vi "Begin.vi"(8 "error in":errorcluster) -> (0 "error out":errorcluster)   [LabVIEW 2015]
doc: "Called before other user functions, this VI is expected to open initial I/O refnums, load in file data, and do all program initialization. Notice that the <B>error out</B> terminal is simply used for data flow. Wiring it to other structures or subVIs ensures that this VI runs first."
uses:
  <vilib>/Rock Robotics/WPI/DriverStation/WPI_DriverStationRobotMode2.ctl
  <vilib>/Rock Robotics/WPI/Joystick/WPI_JoystickDeviceEnum.ctl
  <vilib>/Rock Robotics/SystemInterfaces/DIO/FPGA_DIOChannel.ctl
  <vilib>/Rock Robotics/SystemInterfaces/DIO/FPGA_DIORelayChannel.ctl
  <vilib>/Rock Robotics/WPI/Solenoid/WPI_SolenoidChannel.ctl
  <vilib>/Rock Robotics/SystemInterfaces/DIO/FPGA_DIOPWMChannel.ctl
  <vilib>/Rock Robotics/SystemInterfaces/AI/FPGA_AIGyroChannel.ctl
  <vilib>/Rock Robotics/WPI/SafetyOutput/WPI_SafetyOutputConfigMenu.ctl
  <vilib>/Rock Robotics/SystemInterfaces/spilib/spi_bus.ctl
  Robot Global Data.vi
  <vilib>/Rock Robotics/Network Tables/NT Write String Array.vi
  <vilib>/Rock Robotics/WPI/Switch/WPI_SwitchOpenLimit.vi
  <vilib>/Rock Robotics/WPI/Solenoid/WPI_SolenoidOpenDouble.vi
  <vilib>/Rock Robotics/WPI/Counter/WPI_CounterDigitalInputToDigitalSource.vi
  <vilib>/Rock Robotics/WPI/MotorControl/WPI_MotorControlOpenCANTalonSRX.vi
  <vilib>/Rock Robotics/WPI/Gyro/WPI_GyroAnalogOpen.vi
  <vilib>/Rock Robotics/WPI/Utilities/WPI_GetSetVariantRefNum.vi
  <vilib>/Rock Robotics/WPI/Accelerometer/InternalAccelerometer/WPI_AccelerometerInternalOpen.vi
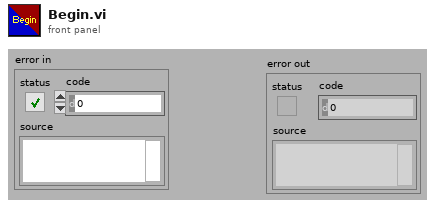
[diagram p1: front panel]
types:
  T1 = typedef "FPGA_AIGyroChannel.ctl" = enum8{"AI 0", "AI 1", "Invalid"}
  T2 = typedef "spi_bus.ctl" = enum16{"SPI On-Board, CS0", "SPI On-Board, CS1", "SPI On-Board, CS2", "SPI On-Board, CS3", "SPI MXP", "Invalid"}
  T3 = typedef "FPGA_DIOChannel.ctl" = enum8{"DIO 0", "DIO 1", "DIO 2", "DIO 3", "DIO 4", "DIO 5", "DIO 6", "DIO 7", "DIO 8", "DIO 9", "DIO MXP 0", "DIO MXP 1", "DIO MXP 2", "DIO MXP 3", "DIO MXP 4", "DIO MXP 5", "DIO MXP 6", "DIO MXP 7", "DIO MXP 8", "DIO MXP 9", "DIO MXP 10", "DIO MXP 11", "DIO MXP 12", "DIO MXP 13", "DIO MXP 14", "DIO MXP 15", "Invalid"}
  T4 = typedef "FPGA_DIOPWMChannel.ctl" = enum8{"PWM 0", "PWM 1", "PWM 2", "PWM 3", "PWM 4", "PWM 5", "PWM 6", "PWM 7", "PWM 8", "PWM 9", "PWM MXP 0", "PWM MXP 1", "PWM MXP 2", "PWM MXP 3", "PWM MXP 4", "PWM MXP 5", "PWM MXP 6", "PWM MXP 7", "PWM MXP 8", "PWM MXP 9", "Invalid"}
  T5 = typedef "WPI_SolenoidChannel.ctl" = enum8{"Solenoid 0", "Solenoid 1", "Solenoid 2", "Solenoid 3", "Solenoid 4", "Solenoid 5", "Solenoid 6", "Solenoid 7", "Invalid"}
  T6 = typedef "FPGA_DIORelayChannel.ctl" = enum8{"Relay 0", "Relay 1", "Relay 2", "Relay 3", "Invalid"}
  T7 = typedef "WPI_JoystickDeviceEnum.ctl" = enum16{"USB 0", "USB 1", "USB 2", "USB 3", "USB 4", "USB 5"}
  T8 = typedef "WPI_DriverStationRobotMode2.ctl" = enum16{"Autonomous Disabled", "Autonomous Enabled", "Teleop Disabled", "Teleop Enabled", "Disconnected", "Finish", "Test Disabled", "Test Enabled", "Emergency Stopped"}
  T9 = typedef "WPI_SafetyOutputConfigMenu.ctl" = enum16{"Enable", "Disable"}
  T10 = typedef "WPI_AccelerometerDevRef.ctl" = cluster{"DevStatus":errorcluster, "Scaling":T11, "Analog Channels":T12, "I2C Bus":T14, "SPI Bus":T2, "Accel Range":T15, "ADXL Axes":T16, "Handle":i32, "Device Address":u8, "Accel Type":enum16{"Analog", "ADXL345 I2C", "ADXL345 SPI", "Internal", "ADXL362 SPI"}}
  T11 = typedef "WPI_AccelerometerScaling.ctl" = cluster{"Gain (VoltsPerG)":dbl, "Center Voltage":dbl}
  T12 = typedef "WPI_AccelerometerAnalogChannels.ctl" = cluster{"X-Axis":T13, "Y-Axis":T13, "Z-Axis":T13}
  T13 = typedef "FPGA_AIChannel.ctl" = enum8{"AI 0", "AI 1", "AI 2", "AI 3", "AI MXP 0", "AI MXP 1", "AI MXP 2", "AI MXP 3", "Invalid"}
  T14 = typedef "i2c_bus.ctl" = enum16{"I2C On-Board", "I2C MXP", "Invalid"}
  T15 = typedef "ADXL345 Range.ctl" = u8
  T16 = typedef "WPI_AccelerometerADXL345 Axes.ctl" = cluster{"X-Axis":bool, "Y-Axis":bool, "Z-Axis":bool}
  T17 = typedef "WPI_CompressorDevRef.ctl" = cluster{"DevStatus":errorcluster, "Pneumatics Control Module":u8}
  T18 = typedef "WPI_MotorControlDeviceRef.ctl" = cluster{"DeviceStatus":errorcluster, "Type":T19, "PWM":cluster{"PWM Channel":T4, "DeadBand":T20}, "CAN":cluster{"Device Number":u8, "Control Mode":T21, "Semaphore":T22, "Max Vout":dbl, "TalonSRX Control Mode":T23}, "Invert":bool}
  T19 = typedef "WPI_MotorControlType.ctl" = enum16{"PWM", "CAN", "CANTalonSRX"}
  T20 = typedef "WPI_PWMDeadband.ctl" = cluster{"Name":string, "maxPositivePwm":i32, "minPositivePwm":i32, "centerPwm":i32, "maxNegativePwm":i32, "minNegativePwm":i32, "angularRange":u16}
  T21 = typedef "WPI_CANJaguar_ControlMode.ctl" = enum8{"Percent VBus", "Current", "Speed", "Position", "Voltage"}
  T22 = typedef "Semaphore RefNum" = refnum<k1>
  T23 = typedef "WPI_CANTalonSRX_APIControlMode.ctl" = enum8{"Percent VBus", "Speed", "Position", "Slave", "Unchanged / Invalid", "Voltage Compensation", "Current", "Motion Profile"}
  T24 = typedef "WPI_JoystickDevRef.ctl" = cluster{"Device":T7}
  T25 = typedef "WPI_DigitalInputDevRef.ctl" = cluster{"DevStatus":errorcluster, "DIO Channel":T3}
  T26 = typedef "WPI_SwitchDevRef.ctl" = cluster{"DevStatus":errorcluster, "DIO Channel":T3, "CntIndex":T27, "Normally Closed":bool}
  T27 = typedef "FPGA_CounterCtrSystemIndex.ctl" = enum8{"Ctr 0", "Ctr 1", "Ctr 2", "Ctr 3", "Ctr 4", "Ctr 5", "Ctr 6", "Ctr 7", "Invalid"}
  T28 = typedef "WPI_ServoDeviceRef.ctl" = cluster{"DeviceStatus":errorcluster, "PWM Channel":T4, "DeadBand":T20}
  T29 = typedef "WPI_RelayDevRef.ctl" = cluster{"DevStatus":errorcluster, "Relay Channel":T6, "Relay Direction":T30}
  T30 = typedef "WPI_RelayDirection.ctl" = enum16{"Both directions", "Forward only", "Reverse only"}
  T31 = typedef "WPI_SolenoidDevRef.ctl" = cluster{"DevStatus":errorcluster, "Pneumatics Control Module":u8, "Forward Solenoid Channel":T5, "Reverse Solenoid Channel":T5}
  T32 = typedef "FPGA_CounterEncoderSourceConvertionLVSourceType.ctl" = cluster{"DevStatus":errorcluster, "AnalogTriggerMode?":bool, "DigitalMode":cluster{"DIO Channel":T33}, "AnalogTriggerMode":cluster{"AnalogTriggerIndex":T34, "OutputType":T35}}
  T33 = typedef "FPGA_DIODigitalSourceChannel.ctl" = enum8{"DIO 0", "DIO 1", "DIO 2", "DIO 3", "DIO 4", "DIO 5", "DIO 6", "DIO 7", "DIO 8", "DIO 9", "DIO MXP 0", "DIO MXP 1", "DIO MXP 2", "DIO MXP 3", "DIO MXP 4", "DIO MXP 5", "DIO MXP 6", "DIO MXP 7", "DIO MXP 8", "DIO MXP 9", "DIO MXP 10", "DIO MXP 11", "DIO MXP 12", "DIO MXP 13", "DIO MXP 14", "DIO MXP 15", "Disabled"}
  T34 = typedef "FPGA_AnalogTriggerIndex.ctl" = enum8{"Trig 0", "Trig 1", "Trig 2", "Trig 3", "Trig 4", "Trig 5", "Trig 6", "Trig 7", "Invalid"}
  T35 = typedef "FPGA_AnalogTriggerOutType.ctl" = enum16{"InWindow", "TriggerState", "Rising", "Falling"}
  T36 = typedef "WPI_GyroDevRef.ctl" = cluster{"DevStatus":errorcluster, "Analog Channel":T13, "Offset":dbl, "Gain (VoltsPerDegree/Second)":dbl, "Gyro Type":enum16{"Analog", "XRS450"}, "Handle":i32, "SPI Bus":T2, "Device Found":bool, "Sample Rate":dbl, "Calibrate On Open":bool}
  T37 = typedef "WPI_EncoderDevRef.ctl" = cluster{"DevStatus":errorcluster, "EncoderIndex":T38, "CounterIndex":T27, "DistancePerCount":dbl, "Decoding Type":T39}
  T38 = typedef "FPGA_EncoderIdx.ctl" = enum8{"Enc 0", "Enc 1", "Enc 2", "Enc 3", "Enc 4", "Enc 5", "Enc 6", "Enc 7", "Invalid"}
  T39 = typedef "WPI_EncoderType.ctl" = enum16{"1x", "2x", "4x"}
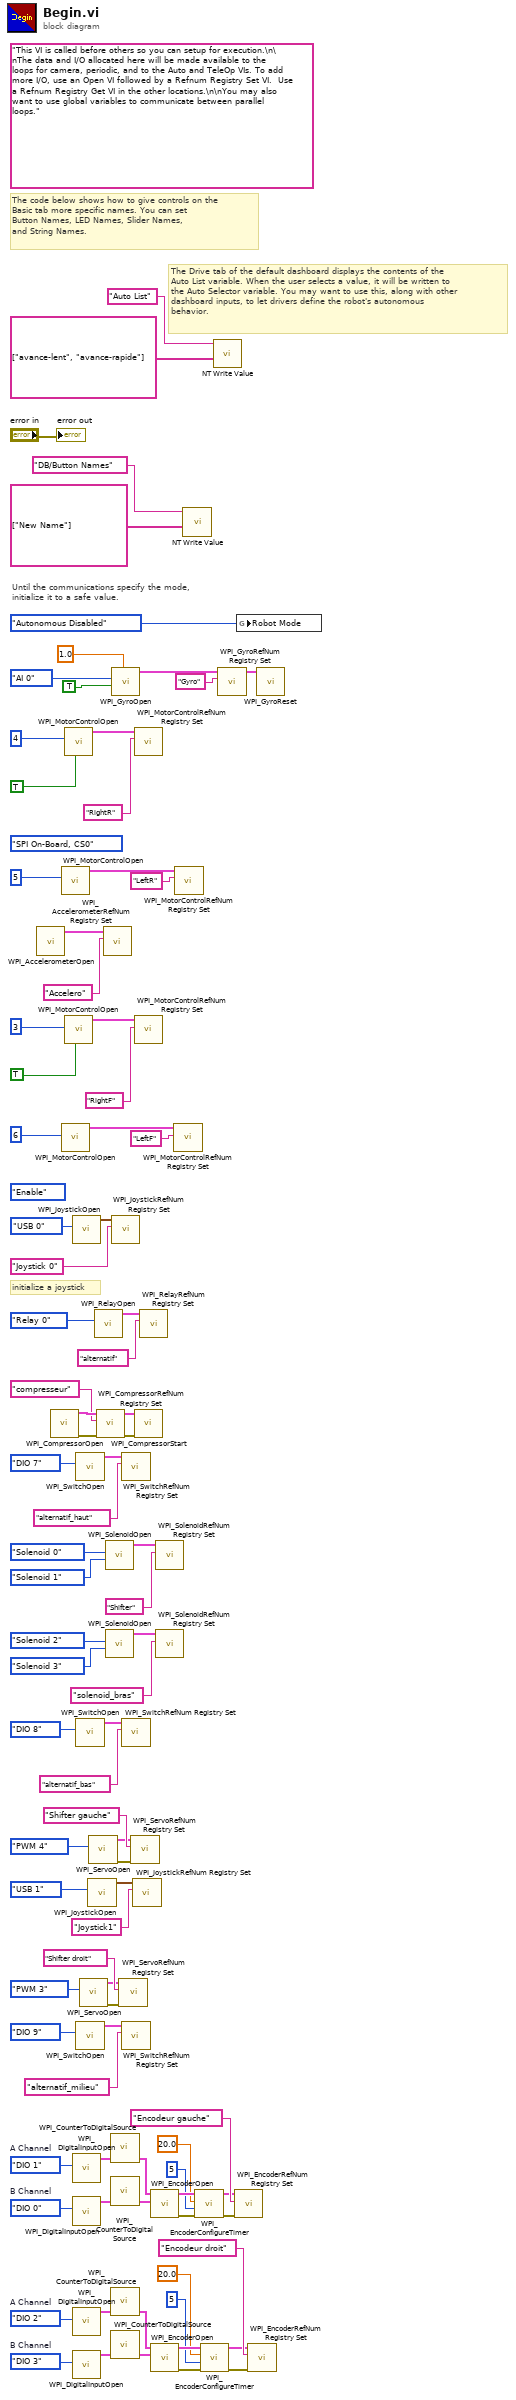
[diagram p0: block diagram]
diagram:
  (unwired) spi_bus."SPI On-Board, CS0" ("SPI Bus")
  w41 = FPGA_DIOChannel."DIO 0"  # B Channel
  w40 = FPGA_DIOChannel."DIO 1"  # A Channel
  w48 = FPGA_DIOChannel."DIO 3"  # B Channel
  w47 = FPGA_DIOChannel."DIO 2"  # A Channel
  (unwired) WPI_SafetyOutputConfigMenu."Enable" ("mode")
  (unwired) "This VI is called before others so you can setup for execution.\n\nThe data and I/O allocated here will be made available to the loops for camera, periodic, and to the Auto and TeleOp VIs. To add more I/O, use an Open VI followed by a Refnum Registry Set VI.  Use a Refnum Registry Get VI in the other locations.\n\nYou may also want to use global variables to communicate between parallel loops."
  # "The Drive tab of the default dashboard displays the contents of the\nAuto List variable. When the user selects a value, it will be written to\nthe Auto Selector variable. You may want to use this, along with other\ndashboard inputs, to let drivers define the robot's autonomous\nbehavior."
  # "The code below shows how to give controls on the\nBasic tab more specific names. You can set\nButton Names, LED Names, Slider Names,\nand String Names."
  # "initialize a joystick"
  # "Until the communications specify the mode,\ninitialize it to a safe value."
  n1 = call-poly <vilib>:"WPI_AccelerometerOpen.vi"() -> ("AccelerometerDevRef"=w28:T10)  [unwired: 10 in, 1 out]
  n2 = call <vilib>:"WPI_CompressorOpen.vi"() -> ("CompressorDevRef"=w60:T17, "error out"=w61:errorcluster)  [unwired: 14 in]
  n3 = call-poly <vilib>:"WPI_MotorControlOpen.vi"("Device Number"=u8 5) -> ("MotorControlDeviceRef"=w9:T18)  [unwired: 9 in, 1 out]
  n4 = call-poly <vilib>:"WPI_MotorControlOpen.vi"("Device Number"=u8 6) -> ("MotorControlDeviceRef"=w7:T18)  [unwired: 9 in, 1 out]
  n5 = call-poly <vilib>:"WPI_MotorControlOpen.vi"("Invert"=TRUE, "Device Number"=u8 4) -> ("MotorControlDeviceRef"=w10:T18)  [unwired: 8 in, 1 out]
  n6 = call-poly <vilib>:"WPI_MotorControlOpen.vi"("Invert"=TRUE, "Device Number"=u8 3) -> ("MotorControlDeviceRef"=w8:T18)  [unwired: 8 in, 1 out]
  n7 = call <vilib>:"WPI_JoystickOpen.vi"("JoystickDevice"=WPI_JoystickDeviceEnum."USB 0") -> ("JoystickDevRef"=w91:T24)  [unwired: 10 in]
  n8 = call <vilib>:"WPI_DigitalInputOpen.vi"("DIO Channel"=w40) -> ("DigitalInputDevRef"=w37:T25)  [unwired: 1 in, 9 out]
  n9 = call <vilib>:"WPI_DigitalInputOpen.vi"("DIO Channel"=w41) -> ("DigitalInputDevRef"=w38:T25)  [unwired: 1 in, 9 out]
  n10 = call <vilib>:"WPI_DigitalInputOpen.vi"("DIO Channel"=w47) -> ("DigitalInputDevRef"=w44:T25)  [unwired: 1 in, 9 out]
  n11 = call <vilib>:"WPI_DigitalInputOpen.vi"("DIO Channel"=w48) -> ("DigitalInputDevRef"=w45:T25)  [unwired: 1 in, 9 out]
  n12 = call-poly <vilib>:"WPI_SwitchOpen.vi"("DIO Channel"=FPGA_DIOChannel."DIO 7") -> ("SwitchDevRef"=w81:T26)  [unwired: 9 in, 1 out]
  n13 = call-poly <vilib>:"WPI_SwitchOpen.vi"("DIO Channel"=FPGA_DIOChannel."DIO 8") -> ("SwitchDevRef"=w78:T26)  [unwired: 9 in, 1 out]
  n14 = call-poly <vilib>:"WPI_SwitchOpen.vi"("DIO Channel"=FPGA_DIOChannel."DIO 9") -> ("SwitchDevRef"=w71:T26)  [unwired: 9 in, 1 out]
  n15 = call <vilib>:"WPI_ServoOpen.vi"("PWM Channel"=FPGA_DIOPWMChannel."PWM 3" ("Front Left Motor")) -> ("error out"=w51:errorcluster, "ServoDeviceRef"=w54:T28)  [unwired: 9 in]
  n16 = call <vilib>:"WPI_JoystickOpen.vi"("JoystickDevice"=WPI_JoystickDeviceEnum."USB 1") -> ("JoystickDevRef"=w75:T24)  [unwired: 10 in]
  n17 = call <vilib>:"WPI_ServoOpen.vi"("PWM Channel"=FPGA_DIOPWMChannel."PWM 4" ("Front Left Motor")) -> ("error out"=w52:errorcluster, "ServoDeviceRef"=w53:T28)  [unwired: 9 in]
  n18 = call <vilib>:"WPI_RelayOpen.vi"("Relay Channel"=FPGA_DIORelayChannel."Relay 0") -> ("RelayDevRef"=w70:T29)  [unwired: 9 in, 1 out]
  n19 = call <vilib>:"WPI_CompressorRefNum Registry Set.vi"("error in (no error)"=w61, "refnum name"="compresseur", "CompressorDevRef"=w60) -> ("error out"=w57:errorcluster, "CompressorDevRef"=w59:T17)  [unwired: 7 in]
  n20 = call <vilib>:"WPI_AccelerometerRefNum Registry Set.vi"("refnum name"="Accelero", "AccelerometerDevRef"=w28) -> ()  [unwired: 8 in, 2 out]
  n21 = call-poly <vilib>:"WPI_SolenoidOpen.vi"("Reverse Solenoid Channel"=WPI_SolenoidChannel."Solenoid 1", "Forward Solenoid Channel"=WPI_SolenoidChannel."Solenoid 0") -> ("SolenoidDevRef"=w64:T31)  [unwired: 8 in, 1 out]
  n22 = call-poly <vilib>:"WPI_SolenoidOpen.vi"("Reverse Solenoid Channel"=WPI_SolenoidChannel."Solenoid 3", "Forward Solenoid Channel"=WPI_SolenoidChannel."Solenoid 2") -> ("SolenoidDevRef"=w68:T31)  [unwired: 8 in, 1 out]
  n23 = call-poly <vilib>:"WPI_CounterToDigitalSource.vi"("DigitalInputDevRef"=w37) -> ("Digital Source"=w36:T32)  [unwired: 6 out]
  n24 = call-poly <vilib>:"WPI_CounterToDigitalSource.vi"("DigitalInputDevRef"=w38) -> ("Digital Source"=w39:T32)  [unwired: 6 out]
  n25 = call-poly <vilib>:"WPI_CounterToDigitalSource.vi"("DigitalInputDevRef"=w44) -> ("Digital Source"=w43:T32)  [unwired: 6 out]
  n26 = call-poly <vilib>:"WPI_CounterToDigitalSource.vi"("DigitalInputDevRef"=w45) -> ("Digital Source"=w46:T32)  [unwired: 6 out]
  n27 = call-poly <vilib>:"WPI_GyroOpen.vi"("Calibration Time (s)"=1.0, "Calibrate On Open"=TRUE, "Analog Channel"=FPGA_AIGyroChannel."AI 0") -> ("GyroDevRef"=w33:T36)  [unwired: 6 in, 2 out]
  n28 = call <vilib>:"WPI_JoystickRefNum Registry Set.vi"("refnum name"="Joystick 0", "JoystickDevRef"=w91) -> ()  [unwired: 8 in, 2 out]
  n29 = call <vilib>:"WPI_ServoRefNum Registry Set.vi"("error in (no error)"=w51, "refnum name"="Shifter droit", "ServoDeviceRef"=w54) -> ()  [unwired: 7 in, 2 out]
  n30 = call <vilib>:"WPI_SwitchRefNum Registry Set.vi"("refnum name"="alternatif_haut", "SwitchDevRef"=w81) -> ()  [unwired: 8 in, 2 out]
  n31 = call <vilib>:"WPI_SwitchRefNum Registry Set.vi"("refnum name"="alternatif_bas", "SwitchDevRef"=w78) -> ()  [unwired: 8 in, 2 out]
  n32 = call <vilib>:"WPI_SwitchRefNum Registry Set.vi"("refnum name"="alternatif_milieu", "SwitchDevRef"=w71) -> ()  [unwired: 8 in, 2 out]
  n33 = call <vilib>:"WPI_ServoRefNum Registry Set.vi"("error in (no error)"=w52, "refnum name"="Shifter gauche", "ServoDeviceRef"=w53) -> ()  [unwired: 7 in, 2 out]
  n34 = call <vilib>:"WPI_JoystickRefNum Registry Set.vi"("refnum name"="Joystick1", "JoystickDevRef"=w75) -> ()  [unwired: 8 in, 2 out]
  n35 = call <vilib>:"WPI_MotorControlRefNum Registry Set.vi"("refnum name"="RightR", "MotorControlDevRef"=w10) -> ()  [unwired: 8 in, 2 out]
  n36 = call <vilib>:"WPI_MotorControlRefNum Registry Set.vi"("refnum name"="RightF", "MotorControlDevRef"=w8) -> ()  [unwired: 8 in, 2 out]
  n37 = call <vilib>:"WPI_CompressorStart.vi"("error in (no error)"=w57, "CompressorDevRef"=w59) -> ()  [unwired: 8 in, 2 out]
  n38 = call <vilib>:"WPI_RelayRefNum Registry Set.vi"("refnum name"="alternatif", "RelayDevRef"=w70) -> ()  [unwired: 8 in, 2 out]
  n39 = call <vilib>:"WPI_EncoderOpen.vi"("BSource"=w39, "ASource"=w36) -> ("error out"=w21:errorcluster, "EncoderDevRef"=w26:T37)  [unwired: 6 in, 2 out]
  n40 = call <vilib>:"WPI_EncoderOpen.vi"("BSource"=w46, "ASource"=w43) -> ("error out"=w18:errorcluster, "EncoderDevRef"=w20:T37)  [unwired: 6 in, 2 out]
  n41 = call <vilib>:"WPI_SolenoidRefNum Registry Set.vi"("refnum name"="Shifter", "SolenoidDevRef"=w64) -> ()  [unwired: 8 in, 2 out]
  n42 = call <vilib>:"WPI_SolenoidRefNum Registry Set.vi"("refnum name"="solenoid_bras", "SolenoidDevRef"=w68) -> ()  [unwired: 8 in, 2 out]
  n43 = call <vilib>:"WPI_MotorControlRefNum Registry Set.vi"("refnum name"="LeftF", "MotorControlDevRef"=w7) -> ()  [unwired: 8 in, 2 out]
  n44 = call <vilib>:"WPI_MotorControlRefNum Registry Set.vi"("refnum name"="LeftR", "MotorControlDevRef"=w9) -> ()  [unwired: 8 in, 2 out]
  n45 = call-poly <vilib>:"NT Write Value.vi"("String Array"=string[] ["New Name"], "Name"="DB/Button Names") -> ()  [unwired: 9 in, 1 out]
  n46 = call <vilib>:"WPI_EncoderConfigureTimer.vi"("error in (no error)"=w21, "Number Samples to Average"=u8 5, "Minimum Rate"=20.0, "EncoderDevRef"=w26) -> ("error out"=w22:errorcluster, "EncoderDevRef"=w25:T37)  [unwired: 6 in]
  n47 = call <vilib>:"WPI_EncoderConfigureTimer.vi"("error in (no error)"=w18, "Number Samples to Average"=u8 5, "Minimum Rate"=20.0, "EncoderDevRef"=w20) -> ("error out"=w17:errorcluster, "EncoderDevRef"=w19:T37)  [unwired: 6 in]
  n48 = call-poly <vilib>:"NT Write Value.vi"("String Array"=string[] ["avance-lent", "avance-rapide"], "Name"="Auto List") -> ()  [unwired: 9 in, 1 out]
  n49 = call <vilib>:"WPI_GyroRefNum Registry Set.vi"("refnum name"="Gyro", "GyroDevRef"=w33) -> ("GyroDevRef"=w29:T36)  [unwired: 8 in, 1 out]
  n50 = call <vilib>:"WPI_EncoderRefNum Registry Set.vi"("error in (no error)"=w22, "refnum name"="Encodeur gauche", "EncoderDevRef"=w25) -> ()  [unwired: 7 in, 2 out]
  n51 = global write "Robot Global Data.vi" "Robot Mode"(WPI_DriverStationRobotMode2."Autonomous Disabled" ("Robot Mode")) -> ()
  n52 = call <vilib>:"WPI_EncoderRefNum Registry Set.vi"("error in (no error)"=w17, "refnum name"="Encodeur droit", "EncoderDevRef"=w19) -> ()  [unwired: 7 in, 2 out]
  n53 = call <vilib>:"WPI_GyroReset.vi"("GyroDevRef"=w29) -> ()  [unwired: 9 in, 2 out]
  "error out" <- "error in"
